vi "VM_ProjetoV3.vi"() -> ()   [LabVIEW 2016]
panel:
  in  "Origin Pixel":dbl[](array[numeric])
  in  "Step":sgl=0.29742944
  in  "Cut Limit":dbl=55.0 format="%#_13g"
  out "Dobrao":bool
  out "Passa Vez":bool
  out "place pos Norm":dbl[](array[numeric])
  out "pick pos Norm":dbl[](array[numeric])
  out "place angle":dbl
  out "pick angle":dbl
  out "Image Out 2":T1(plugin-control)
  in  "Source Mao":path=path "C:/Users/Alexandre/Documents/LabView Projects/Projeto/Source/Others/base1.png"
  out "Image Out":T1(plugin-control)
  in  "Source Mesa":path=path "C:/Users/Alexandre/Documents/LabView Projects/Projeto/Source/Base"
  # "x 91\ny 176"
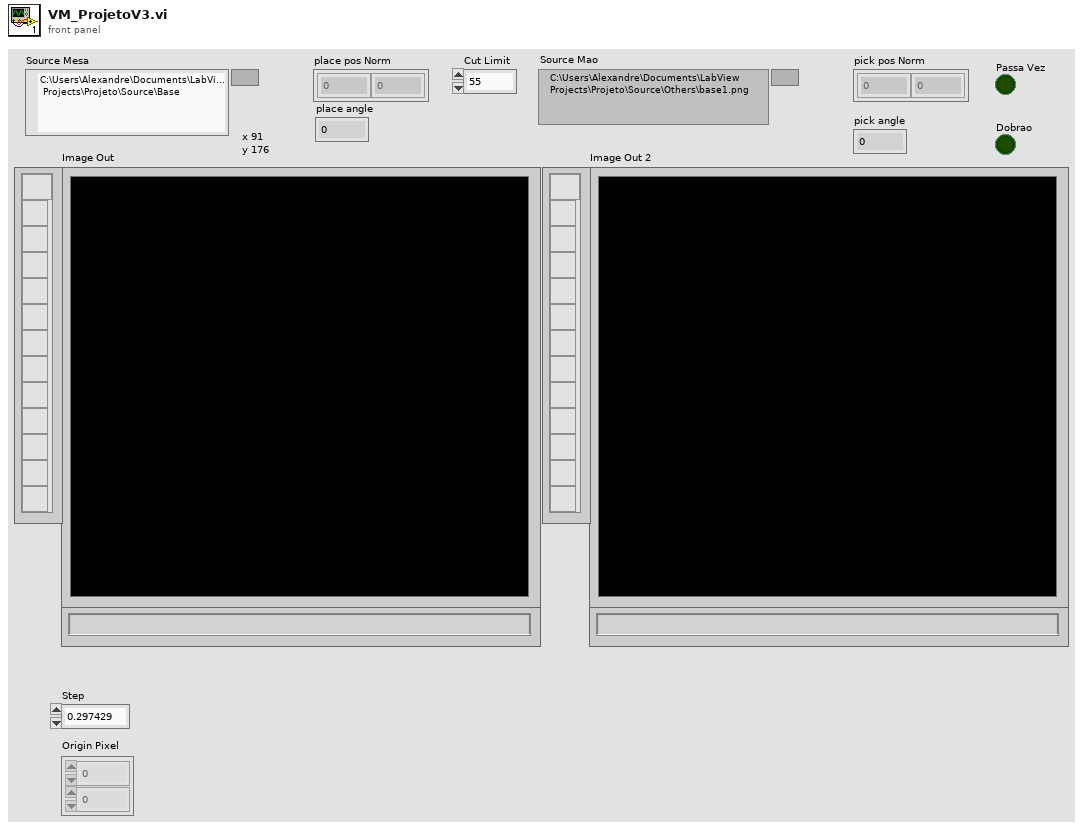
[diagram p1: front panel]
types:
  T1 = typedef "IMAQ Image.ctl" = refnum<image>
  T2 = cluster{"Position":cluster{"x":sgl, "y":sgl}, "Angle":sgl, "Scale":sgl, "Score":sgl, "Bounding Box":cluster{"x":sgl, "y":sgl}[]}[]
  T3 = typedef "ROI Descriptor" = cluster{"Global Rectangle":i32[], "Contours":cluster{"ID":enum32{"External", "Internal"}, "Type":u32, "Coordinates":i32[]}[]}
  T4 = cluster{"Centro Peça":dbl[], "Centros Númeors":dbl[][], "Números":u8[], "ROI Números":T3[]}[]
  T5 = cluster{"Centro Peça":dbl[], "Centros Númeors":dbl[][], "Números":u8[], "ROI Números":T3[]}
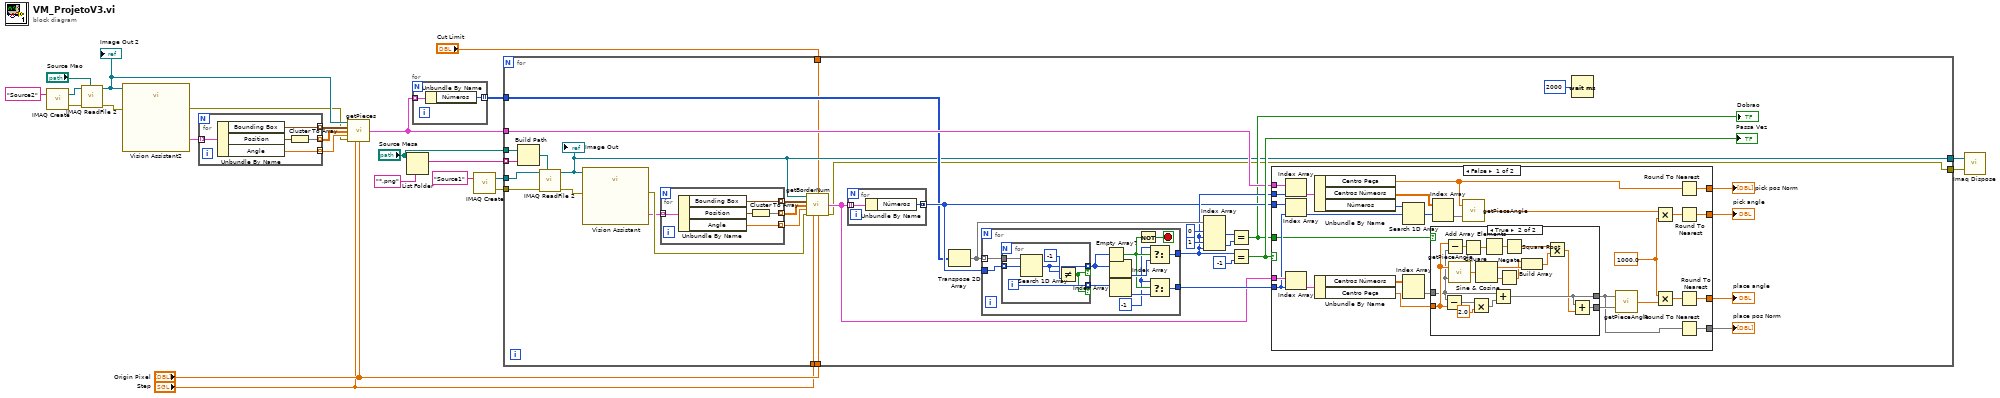
[diagram p0: block diagram]
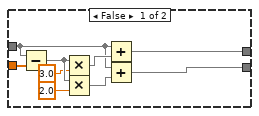
[diagram p2: hidden frame]
diagram:
  n1 = call "IMAQ Create"("Image Name"="Source2") -> ("New Image"=w17:T1, "error out"=w16:errorcluster)  [unwired: 4 in]
  n2 = call "IMAQ ReadFile 2"("File Path"="Source Mao", "error in (no error)"=w16, "Image"=w17) -> ("error out"=w14:errorcluster, "Image Out"=w8:T1)  [unwired: 4 in, 3 out]
  "Image Out 2" <- w8
  n3 = call "Vision Assistant2"("Image In"=w8, "error in"=w14) -> ("Matches (Pattern Matching 1)"=w3:T2, "error out"=w5:errorcluster)  [unwired: 23 in, 1 out]
  n4 = for {
    tunnel: [w29] -> w12 mode=indexing
    tunnel: [w28] -> w13 mode=indexing
    tunnel: [w25] -> w11 mode=indexing
    tunnel: w3 -> [w27] mode=indexing
    n5 = Unbundle By Name(w27) -> ("Bounding Box"=w28:cluster{"x":sgl, "y":sgl}[], "Position"=w26:cluster{"x":sgl, "y":sgl}, "Angle"=w25:sgl)
    n6 = Cluster To Array(cluster=w26) -> (array=w29:sgl[])
  }
  n7 = call "getPieces.vi"("Refnum in"=w8, "Bounding Box"=w13, "Position"=w12, "Angle"=w11, "error in (no error)"=w5, "Step"="Step", "Origin Pixel"="Origin Pixel") -> ("Data Pieces"=w10:T4)  [unwired: 6 in, 2 out]
  n8 = List Folder(path="Source Mesa", pattern="*.png") -> (filenames=w19:string[])  [unwired: 2 in, 3 out]
  n9 = for {
    tunnel: w10 -> [w31] mode=indexing
    tunnel: [w30] -> w9 mode=indexing
    n10 = Unbundle By Name(w31) -> ("Números"=w30:u8[])
  }
  n11 = call "IMAQ Create"("Image Name"="Source1") -> ("New Image"=w21:T1, "error out"=w20:errorcluster)  [unwired: 4 in]
  n12 = for {
    tunnel: w19 -> [w66] mode=indexing
    tunnel: "Source Mesa" -> [w65]
    tunnel: w21 -> [w64]
    tunnel: w20 -> [w61]
    tunnel: [w41] -> w7
    tunnel: w10 -> [w44]
    tunnel: w9 -> [w43]
    tunnel: [w40] -> w6
    tunnel: "Cut Limit" -> [w39]
    tunnel: "Step" -> [w37]
    tunnel: "Origin Pixel" -> [w36]
    n13 = Build Path(base path=w65, name or relative path=w66) -> (appended path=w63:path)
    n14 = call "IMAQ ReadFile 2"("File Path"=w63, "error in (no error)"=w61, "Image"=w64) -> ("error out"=w62:errorcluster, "Image Out"=w41:T1)  [unwired: 4 in, 3 out]
    "Image Out" <- w41
    n15 = call "Vision Assistant"("Image In"=w41, "error in"=w62) -> ("Matches (Pattern Matching 1)"=w38:T2, "error out"=w56:errorcluster)  [unwired: 23 in, 1 out]
    n16 = for {
      tunnel: [w143] -> w58 mode=indexing
      tunnel: [w142] -> w59 mode=indexing
      tunnel: [w141] -> w57 mode=indexing
      tunnel: w38 -> [w140] mode=indexing
      n17 = Unbundle By Name(w140) -> ("Bounding Box"=w142:cluster{"x":sgl, "y":sgl}[], "Position"=w144:cluster{"x":sgl, "y":sgl}, "Angle"=w141:sgl)
      n18 = Cluster To Array(cluster=w144) -> (array=w143:sgl[])
    }
    n19 = call "getBorderNum.vi"("Refnum in"=w41, "Cut Limit"=w39, "Bounding Box"=w59, "Position"=w58, "Angle"=w57, "error in (no error)"=w56, "Step"=w37, "Origin Pixel"=w36) -> ("Data Pieces"=w46:T4, "error out"=w40:errorcluster)  [unwired: 5 in, 1 out]
    n20 = for {
      tunnel: w46 -> [w139] mode=indexing
      tunnel: [w138] -> w45 mode=concatenating
      n21 = Unbundle By Name(w139) -> ("Números"=w138:u8[])
    }
    n22 = Transpose 2D Array(2D array=w43) -> (transposed array=w51:u8[][])
    n23 = for {
      tunnel: w51 -> [w131] mode=indexing
      tunnel: w45 -> [w130]
      tunnel: [w122] -> w47
      tunnel: [w121] -> w48
      stop <- w126 stop-if-true
      w123 = -1 ("t")
      n24 = for {
        tunnel: w131 -> [w137]
        tunnel: w130 -> [w136] mode=indexing
        tunnel: [w134] -> w128 mode=indexing if=w132
        tunnel: [w133] -> w127 mode=indexing if=w132
        i -> [w133]
        n25 = Search 1D Array(1D array=w137, element=w136) -> (index of element=w134:i32)  [unwired: 1 in]
        n26 = Not Equal?(x=w134, y=-1) -> (x != y?=w132:bool)
      }
      n27 = Empty Array?(array=w128) -> (empty?=w124:bool)
      n28 = Index Array(array=w128) -> (element=w129:i32)  [unwired: 1 in]
      n29 = Index Array(array=w127) -> (element=w125:i32)  [unwired: 1 in]
      n30 = Not(x=w124) -> (.not. x?=w126:bool)
      n31 = Select(t=w123, s=w124, f=w129) -> (s? t:f=w121:i32)
      n32 = Select(t=w123, s=w124, f=w125) -> (s? t:f=w122:i32)
    }
    n33 = Index Array(array=w51, index (row) #1=0 ("disabled index (row)"), index (col) #1=w48, index (row) #2=1 ("disabled index (row)"), index (col) #2=w48) -> (element #1=w55:u8, element #2=w54:u8)
    n34 = Equal?(x=w55, y=w54) -> (x = y?=w42:bool)
    "Dobrao" <- w42
    n35 = Equal?(x=w48, y=-1) -> (x = y?=w49:bool)
    "Passa Vez" <- w49
    n36 = case shown="False" w49 {
      tunnel: w44 -> [w90 _]
      tunnel: w48 -> [w89 _]
      tunnel: w47 -> [w86 _]
      tunnel: w46 -> [w88 _]
      tunnel: w45 -> [w78 _]
      tunnel: w42 -> [w83 _]
      tunnel: [w72 _] -> w35
      tunnel: [w71 _] -> w34
      tunnel: [w70 _] -> w33
      tunnel: [w69 _] -> w32
      frame False {
        w77 = 1000.0
        n37 = Index Array(array=w90, index=w89) -> (element=w91:T5)
        n38 = Index Array(array=w78, index=w86) -> (element=w85:u8)
        n39 = Index Array(array=w88, index=w86) -> (element=w87:T5)
        n40 = Unbundle By Name(w91) -> ("Centro Peça"=w68:dbl[], "Centros Númeors"=w93:dbl[][], "Números"=w92:u8[])
        n41 = Unbundle By Name(w87) -> ("Centros Númeors"=w80:dbl[][], "Centro Peça"=w79:dbl[])
        n42 = Search 1D Array(1D array=w92, element=w85) -> (index of element=w94:i32)  [unwired: 1 in]
        n43 = Index Array(array=w80) -> (element=w82:dbl[])  [unwired: 2 in]
        n44 = case shown="True" w83 {
          tunnel: w82 -> [w98 w113]
          tunnel: w79 -> [w102 w114]
          tunnel: [w96 w106] -> w81
          tunnel: [w95 w105] -> w67
          frame False {
            n45 = Subtract(x=w98, y=w102) -> (x-y=w101:dbl[])
            n46 = Multiply(x=w101, y=3.0) -> (x*y=w103:dbl[])
            n47 = Multiply(x=w101, y=2.0) -> (x*y=w97:dbl[])
            n48 = Add(x=w98, y=w103) -> (x+y=w95:dbl[])
            n49 = Add(x=w98, y=w97) -> (x+y=w96:dbl[])
          }
          frame True {
            n50 = Subtract(x=w113, y=w114) -> (x-y=w120:dbl[])
            n51 = Subtract(x=w114, y=w113) -> (x-y=w117:dbl[])
            n52 = call "getPieceAngle.vi"("Center Num"=w113, "Center Piece"=w114) -> ("Angle"=w112:dbl)
            n53 = Square(x=w117) -> (x^2=w116:dbl[])
            n54 = Multiply(x=w120, y=2.0) -> (x*y=w118:dbl[])
            n55 = Sine & Cosine(0:w112) -> (1:w110:dbl, 2:w111:dbl)
            n56 = Add Array Elements(numeric array=w116) -> (sum=w115:dbl)
            n57 = Add(x=w113, y=w118) -> (x+y=w105:dbl[])
            n58 = Negate(x=w111) -> (-x=w109:dbl)
            n59 = Square Root(x=w115) -> (sqrt(x)=w107:dbl)
            n60 = Build Array(w109, w110) -> (w108:dbl[])
            n61 = Multiply(x=w107, y=w108) -> (x*y=w104:dbl[])
            n62 = Add(x=w105, y=w104) -> (x+y=w106:dbl[])
          }
        }
        n63 = Index Array(array=w93, index (row)=w94) -> (element=w84:dbl[])  [unwired: 1 in]
        n64 = call "getPieceAngle.vi"("Center Num"=w84, "Center Piece"=w68) -> ("Angle"=w73:dbl)
        n65 = call "getPieceAngle.vi"("Center Num"=w81, "Center Piece"=w67) -> ("Angle"=w74:dbl)
        n66 = Multiply(x=w73, y=w77) -> (x*y=w76:dbl)
        n67 = Multiply(x=w77, y=w74) -> (x*y=w75:dbl)
        n68 = Round To Nearest(number=w68) -> (nearest integer value=w72:dbl[])
        n69 = Round To Nearest(number=w76) -> (nearest integer value=w71:dbl)
        n70 = Round To Nearest(number=w75) -> (nearest integer value=w70:dbl)
        n71 = Round To Nearest(number=w67) -> (nearest integer value=w69:dbl[])
      }
      frame True {
      }
    }
    "pick angle" <- w34
    "pick pos Norm" <- w35
    "place angle" <- w33
    "place pos Norm" <- w32
    n72 = Wait (ms)(milliseconds to wait=u32 2000) -> ()  [unwired: 1 out]
  }
  n73 = call "Imaq Dispose"("Image"=w7, "error in (no error)"=w6) -> ()  [unwired: 4 in, 1 out]
